vi "Write IExporter.vi"(9 "IExporter":refnum<class "IExporter.lvclass">, 11 "CDependencyInspection in":refnum<class "CDependencyInspection.lvclass">) -> (3 "CDependencyInspection out":refnum<class "CDependencyInspection.lvclass">)   [LabVIEW 2020, in "DependencyInspection.lvlib" / "CDependencyInspection.lvclass"]
uses:
  CDependencyInspection.lvclass
  obj/Addons/ExtensionInterfaces.lvlibp/IExporter/IExporter.lvclass
  CDependencyInspection.lvclass/CDependencyInspection.ctl
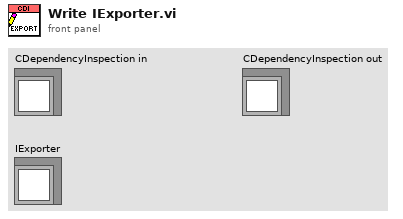
[diagram p1: front panel]
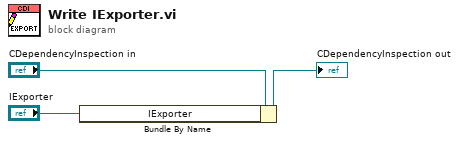
[diagram p0: block diagram]
diagram:
  n1 = Bundle By Name(cluster="CDependencyInspection in", "IExporter"="IExporter") -> (→"CDependencyInspection out":refnum<class "CDependencyInspection.lvclass">)
